vi "Element Init.vi"(7 "VolatusAPI":refnum<class "VolatusAPI.lvclass">, 8 "error in (no error)":errorcluster, 10 "JSON":string, 11 "HistorianCharting in":refnum<class "HistorianCharting.lvclass">) -> (0 "error out":errorcluster, 3 "HistorianCharting out":refnum<class "HistorianCharting.lvclass">)   [LabVIEW 2020, in "VolatusGUIElements.lvlib" / "HistorianCharting.lvclass"]
uses:
  HistorianCharting.lvclass
  Volatus/VolatusAPI/VolatusAPI.lvclass
  HistorianCharting.lvclass/HistorianCharting.ctl
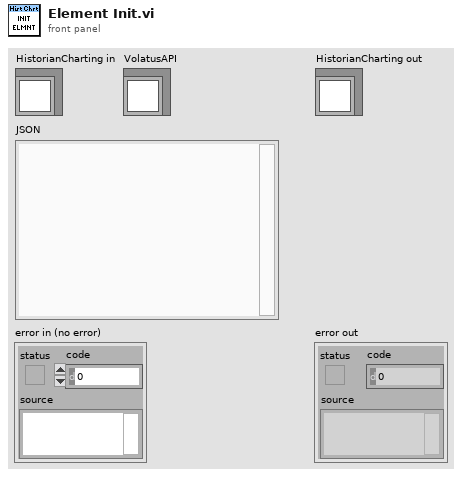
[diagram p1: front panel]
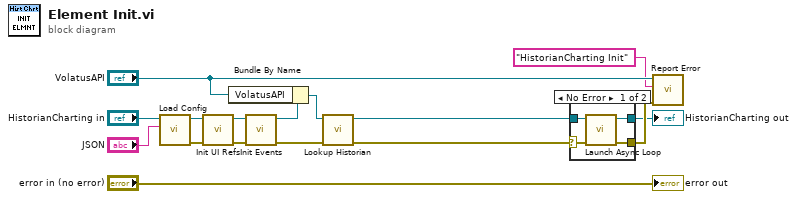
[diagram p0: block diagram]
diagram:
  n1 = call "Load Config.vi"("JSON"="JSON", "HistorianCharting in"="HistorianCharting in") -> ("error out"=w2:errorcluster, "HistorianCharting out"=w3:refnum<class "HistorianCharting.lvclass">)  [unwired: 8 in]
  n2 = call "Init UI Refs.vi"("error in (no error)"=w2, "HistorianCharting in"=w3) -> ("error out"=w15:errorcluster, "HistorianCharting out"=w12:refnum<class "HistorianCharting.lvclass">)  [unwired: 8 in]
  n3 = call "Init Events.vi"("error in (no error)"=w15, "HistorianCharting in"=w12) -> ("error out"=w13:errorcluster, "HistorianCharting out"=w11:refnum<class "HistorianCharting.lvclass">)  [unwired: 8 in]
  n4 = Bundle By Name(cluster=w11, "VolatusAPI"="VolatusAPI") -> (w9:refnum<class "HistorianCharting.lvclass">)
  n5 = call "Lookup Historian.vi"("error in (no error)"=w13, "HistorianCharting in"=w9) -> ("error out"=w10:errorcluster, "HistorianCharting out"=w8:refnum<class "HistorianCharting.lvclass">)  [unwired: 8 in]
  n6 = case shown="No Error" w10 {
    selector: w10 -> [w20 w21]
    tunnel: w8 -> [w19 w22]
    tunnel: [w18 w22] -> w7
    tunnel: [w17 w21] -> w16
    frame No Error {
      n7 = call "Launch Async Loop.vi"("error in (no error)"=w20, "HistorianCharting in"=w19) -> ("error out"=w17:errorcluster, "HistorianCharting out"=w18:refnum<class "HistorianCharting.lvclass">)  [unwired: 8 in]
    }
    frame Error {
    }
  }
  "HistorianCharting out" <- w7
  n8 = call "Report Error.vi"("error in (no error)"=w16, "Context"="HistorianCharting Init", "VolatusAPI in"="VolatusAPI") -> ()  [unwired: 7 in, 2 out]
  "error out" <- "error in (no error)"
